vi "Destroy.vi"(10 "Error":errorcluster, 11 "Self Actor in":refnum<class "Self Actor.lvclass">) -> (0 "error out":errorcluster, 3 "Self Actor out":refnum<class "Self Actor.lvclass">)   [LabVIEW 2021, in "AAM.lvlib" / "Self Actor.lvclass"]
uses:
  Self Actor.lvclass
  C:/PPLs/LabVIEW-Composed-Actor-Model-LVCAM/LabVIEW-Composed-Actor-Model-LVCAM/AAM/AAM/Actor/Actor.lvclass
  Priority Msg EnQ/Priority Msg EnQ.lvclass
  C:/PPLs/LabVIEW-Composed-Actor-Model-LVCAM/LabVIEW-Composed-Actor-Model-LVCAM/AAM/AAM/Msg EnQ/Msg EnQ.lvclass
  Self Actor.lvclass/Self Actor.ctl
  Msgs/Destroy/Destroy Msg/Destroy Msg.lvclass
  C:/PPLs/LabVIEW-Composed-Actor-Model-LVCAM/LabVIEW-Composed-Actor-Model-LVCAM/AAM/AAM/Msg/Msg.lvclass
  Msgs/Last Ack/Last Ack Msg/Last Ack Msg.lvclass
  Nest Msg Send.vi
  Call Msg Send.vi
  Msg Q/Msg Q.lvclass
  C:/PPLs/LabVIEW-Composed-Actor-Model-LVCAM/LabVIEW-Composed-Actor-Model-LVCAM/AAM/AAM/Priority Msg EnQ/Priority Msg EnQ.lvclass
  C:/PPLs/LabVIEW-Composed-Actor-Model-LVCAM/LabVIEW-Composed-Actor-Model-LVCAM/AAM/Msgs/Destroy/Destroy Msg/Destroy Msg.lvclass
  C:/PPLs/LabVIEW-Composed-Actor-Model-LVCAM/LabVIEW-Composed-Actor-Model-LVCAM/AAM/Msgs/Last Ack/Last Ack Msg/Last Ack Msg.lvclass
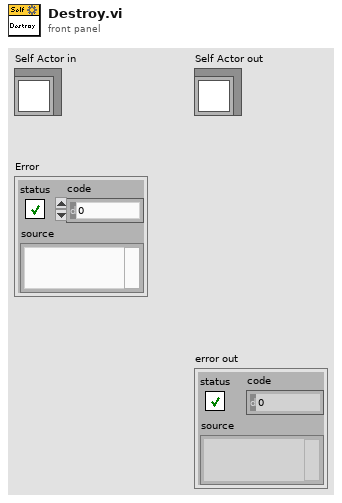
[diagram p1: front panel]
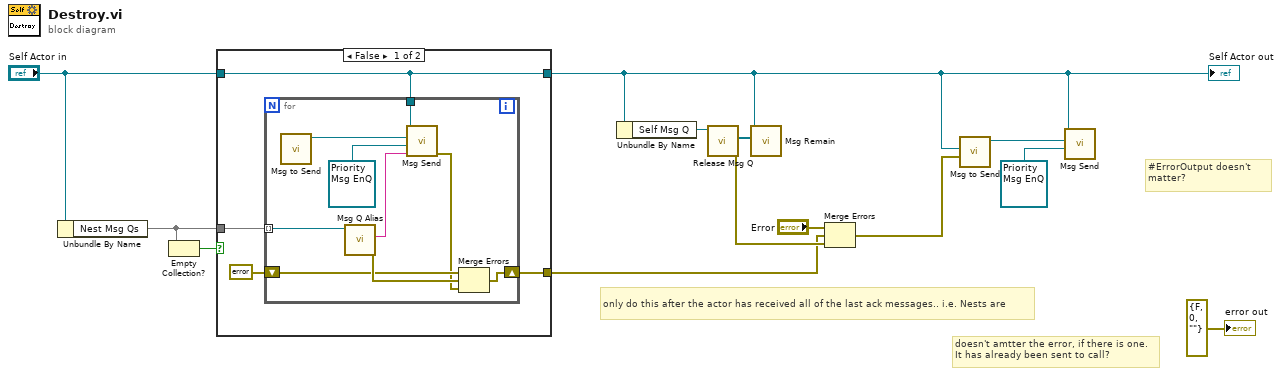
[diagram p0: block diagram]
diagram:
  # "#ErrorOutput doesn't matter?"
  # "doesn't amtter the error, if there is one. It has already been sent to call?"
  # "only do this after the actor has received all of the last ack messages.. i.e. Nests are"
  n1 = Unbundle By Name("Self Actor in") -> ("Nest Msg Qs"=w12:set{refnum<class "Msg Q.lvclass">})
  n2 = Empty Collection?(1:w12) -> (0:w13:bool)
  n3 = case shown="False" w13 {
    tunnel: [w17 w27] -> w3
    tunnel: "Self Actor in" -> [w17 w27]
    tunnel: w12 -> [w16 _]
    tunnel: [w15 _] -> w6
    frame False {
      n4 = for {
        tunnel: w17 -> [w22]
        tunnel: w16 -> [w26] mode=indexing
        shift-right: [w25] -> w15
        shift-left: errorcluster {"status"=FALSE, "code"=0, "source"=""} ("error out") -> [w23]
        n5 = call "Msg to Send.vi"() -> ("Destroy Msg out"=w21:refnum<class "Destroy Msg.lvclass">)  [unwired: 11 in]
        n6 = call "Msg Q Alias.vi"("Msg Q in"=w26) -> ("error out"=w24:errorcluster, "Msg Q Alias"=w19:string)  [unwired: 9 in]
        n7 = call-poly "Msg Send.vi"("Alias"=w19, "Msg EnQ"=refnum<class "Priority Msg EnQ.lvclass"> refnum ("Artifex Actor Model.lvlib:Priority Msg EnQ.lvclass"), "Msg"=w21, "Self Actor in"=w22) -> ("error out"=w18:errorcluster)  [unwired: 7 in]
        n8 = Merge Errors(w23, w24, w18) -> (w25:errorcluster)
      }
    }
    frame True {
    }
  }
  "Self Actor out" <- w3
  n9 = Unbundle By Name(w3) -> ("Self Msg Q"=w9:refnum<class "Msg Q.lvclass">)
  n10 = call "Release Msg Q.vi"("Msg Queue in"=w9) -> ("error out"=w7:errorcluster, "Remaining Elements"=w8:refnum<class "Msg.lvclass">[])  [unwired: 9 in]
  n11 = call-dynamic "Msg Remain.vi"("Remaining Elements"=w8, "Self Actor in"=w3) -> ()  [unwired: 10 in]
  n12 = Merge Errors("Error", w6, w7) -> (w4:errorcluster)
  n13 = call "Msg to Send.vi"("Error"=w4, "Actor"=w3) -> ("Last Ack Msg out"=w2:refnum<class "Last Ack Msg.lvclass">)  [unwired: 9 in]
  n14 = call-poly "Msg Send.vi"("Msg EnQ"=refnum<class "Priority Msg EnQ.lvclass"> refnum ("Artifex Actor Model.lvlib:Priority Msg EnQ.lvclass"), "Msg"=w2, "Self Actor in"=w3) -> ()  [unwired: 8 in, 1 out]
  "error out" <- errorcluster {"status"=FALSE, "code"=0, "source"=""} ("error out")
